vi "visa Init.vi"(8 "error in (no error)":errorcluster, 11 "UI Actor in":refnum<class "UI Actor.lvclass">) -> (0 "error out":errorcluster, 3 "UI Actor out":refnum<class "UI Actor.lvclass">)   [LabVIEW 2020, in "UI Actor.lvlib" / "UI Actor.lvclass"]
uses:
  UI Actor.lvclass
  UI Actor.lvclass/UI Actor.ctl
  Write VISA resource name.vi
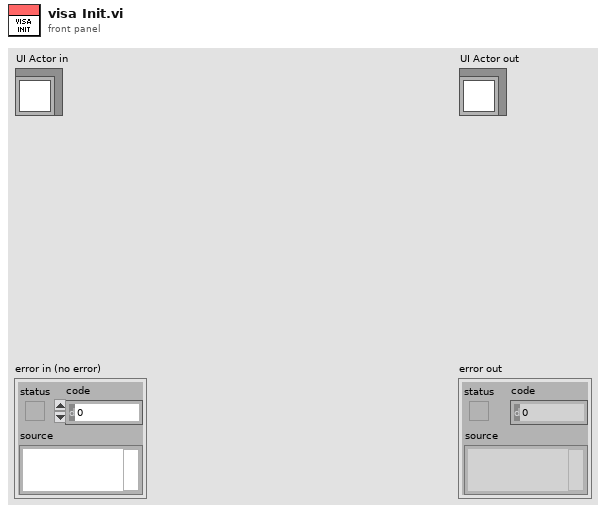
[diagram p1: front panel]
types:
  T1 = enum16{"Write", "Read", "Config", "Reset", "Close"}
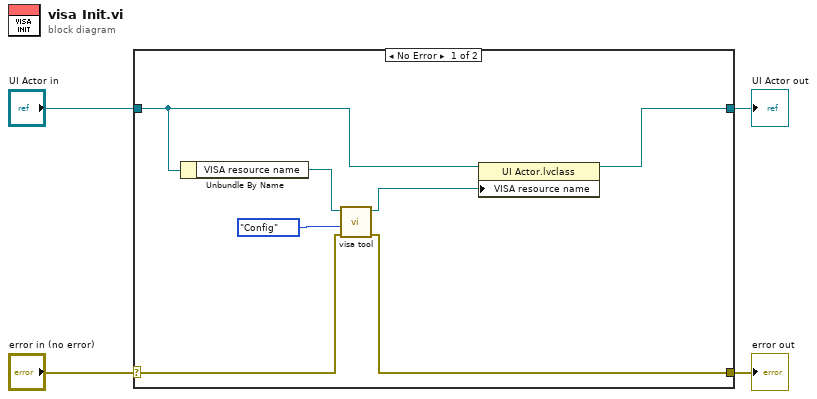
[diagram p0: block diagram]
diagram:
  n1 = case shown="No Error" "error in (no error)" {
    selector: "error in (no error)" -> [w5 w13]
    tunnel: [w6 w13] -> w3
    tunnel: [w10 w12] -> w1
    tunnel: "UI Actor in" -> [w11 w12]
    frame No Error {
      n2 = Unbundle By Name(w11) -> ("VISA resource name"=w9:refnum<visa-resource-name>)
      n3 = call "visa tool.vi"("error in (no error)"=w5, "Opciones"=T1."Config", "VISA com port"=w9) -> ("error out"=w6:errorcluster, "VISA com port 2"=w8:refnum<visa-resource-name>)  [unwired: 6 in, 1 out]
      n4 = property class="UI Actor.lvclass"(reference=w11, "VISA resource name"=w8) -> (reference out=w10:refnum<class "UI Actor.lvclass">)  [unwired: 1 in, 1 out]
    }
    frame Error {
    }
  }
  "error out" <- w3
  "UI Actor out" <- w1
